vi "persistence field value.vi"(1 "Persistent Field In":dbl format="%.2f", 2 "Read/Write this vi":bool) -> (0 "Persistent Field Out":dbl format="%.2f")   [LabVIEW 2019]
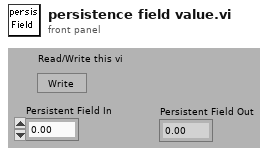
[diagram p1: front panel]
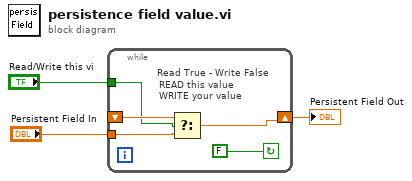
[diagram p0: block diagram]
diagram:
  n1 = while {
    shift-right: [w7] -> w1
    shift-left: _ -> [w6]
    tunnel: "Read/Write this vi" -> [w4]
    tunnel: "Persistent Field In" -> [w8]
    stop <- FALSE continue-if-true
    # "READ this value\nWRITE your value"
    # "Read True - Write False"
    n2 = Select(t=w6, s=w4, f=w8) -> (s? t:f=w7:dbl)
  }
  "Persistent Field Out" <- w1
